vi "P4CMD_Dynam Data Manager.vi"(6 "operation message":string, 7 "function":T2, 8 "error in (no error)":errorcluster, 9 "adv cfg options in":T1, 10 "configuration data":string, 11 "source control reference in":T3) -> (0 "error out":errorcluster, 1 "global commands":string, 2 "initialized?":bool, 3 "source control reference out":T3, 4 "not a refnum?":bool, 5 "adv cfg options out":T1)   [LabVIEW 2017, in "NI_SCC_P4CMD.lvlib"]
uses:
  <vilib>/SourceControl/Providers/P4CMD/NI_SCC_P4CMD.lvlib
  <vilib>/SourceControl/sccapi/SCCAPI Refnum.ctl
  <vilib>/SourceControl/Providers/P4CMD/P4CMD Mgr Functions.ctl
  <vilib>/SourceControl/Providers/P4CMD/P4CMD Advanced Options.ctl
  <vilib>/SourceControl/sccconnsrv/NI_SCC_ConnSrv.lvlib
  <vilib>/SourceControl/sccapi/NI_SCC.lvlib
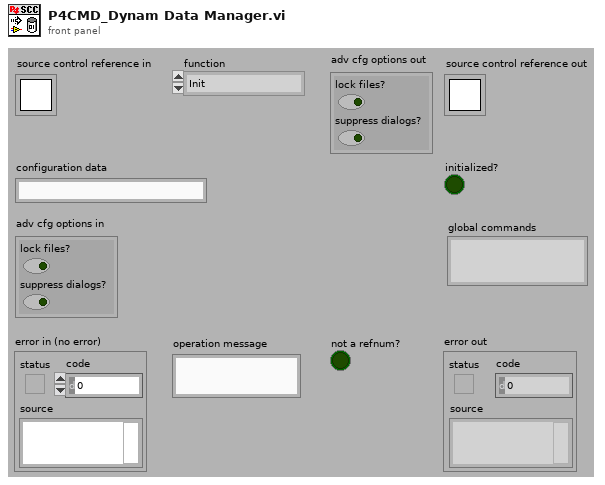
[diagram p1: front panel]
types:
  T1 = typedef "NI_SCC_P4CMD.lvlib/P4CMD Advanced Options.ctl" = cluster{"lock files?":bool, "suppress dialogs?":bool}
  T2 = typedef "NI_SCC_P4CMD.lvlib/P4CMD Mgr Functions.ctl" = enum16{"Init", "Open", "Set Config Opts", "Initialized?", "IsRefValid?", "Get Config Opts", "Get Global Commands", "Close", "Uninit"}
  T3 = typedef "NI_SCC.lvlib/SCCAPI Refnum.ctl" = refnum<k1>
  T4 = typedef "SCCAPI Refnum.ctl" = refnum<k1>
  T5 = typedef "P4CMD Advanced Options.ctl" = cluster{"lock files?":bool, "suppress dialogs?":bool}
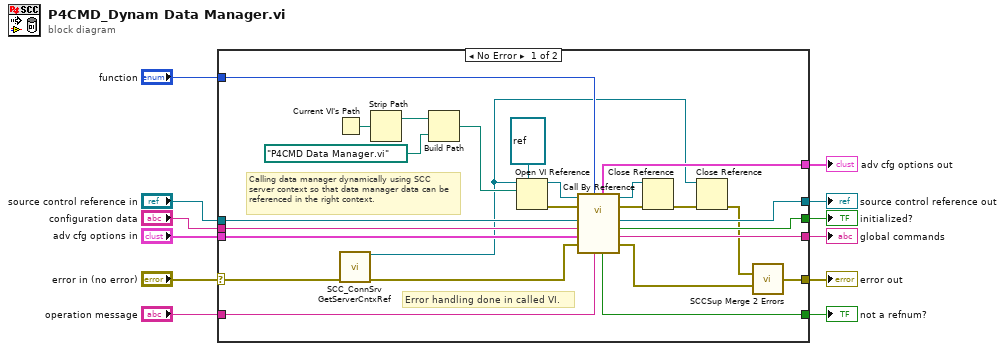
[diagram p0: block diagram]
diagram:
  n1 = case shown="No Error" "error in (no error)" {
    selector: "error in (no error)" -> [w16 w39]
    tunnel: [w38 w39] -> w12
    tunnel: [w37 _] -> w11
    tunnel: "operation message" -> [w36 _]
    tunnel: "configuration data" -> [w35 _]
    tunnel: "function" -> [w34 _]
    tunnel: [w33 _] -> w7
    tunnel: [w32 _] -> w6
    tunnel: [w31 _] -> w5
    tunnel: "source control reference in" -> [w30 _]
    tunnel: [w19 _] -> w3
    tunnel: "adv cfg options in" -> [w18 _]
    frame No Error {
      # "Calling data manager dynamically using SCC server context so that data manager data can be referenced in the right context."
      # "Error handling done in called VI."
      n2 = Current VI's Path() -> (path=w27:path)
      n3 = call <vilib>:"SCC_ConnSrv GetServerCntxRef.vi"("error in (no error)"=w16) -> ("error out"=w17:errorcluster, "SCCServer application reference"=w13:refnum<vi>)  [unwired: 9 in]
      n4 = Strip Path(path=w27) -> (stripped path=w29:path)  [unwired: 1 out]
      n5 = Build Path(base path=w29, name or relative path=path "P4CMD Data Manager.vi") -> (appended path=w26:path)
      n6 = Open VI Reference(type specifier VI Refnum (for type only)=refnum<vi> refnum, application reference (local)=w13, vi path=w26) -> (vi reference=w24:refnum<vi>, error out=w23:errorcluster)  [unwired: 3 in]
      n7 = call-by-ref "?"(reference=w24, error in=w23, "operation message"=w36, "function"=w34, "error in (no error)"=w17, "adv cfg options in"=w18, "configuration data"=w35, "source control reference in"=w30) -> (reference out=w22:refnum<vi>, error out=w21:errorcluster, 0:"error out"=w20:errorcluster, "global commands"=w33:string, "initialized?"=w32:bool, "source control reference out"=w31:T4, "not a refnum?"=w37:bool, "adv cfg options out"=w19:T5)
      n8 = Close Reference(reference=w22, error in (no error)=w21) -> (error out=w15:errorcluster)
      n9 = Close Reference(reference=w13, error in (no error)=w15) -> (error out=w14:errorcluster)
      n10 = call <vilib>:"SCCSup Merge 2 Errors.vi"("Error IO 1"=w14, "Error IO 2"=w20) -> ("Error IO out"=w38:errorcluster)  [unwired: 13 in]
    }
    frame Error {
    }
  }
  "error out" <- w12
  "source control reference out" <- w5
  "global commands" <- w7
  "initialized?" <- w6
  "not a refnum?" <- w11
  "adv cfg options out" <- w3
